vi "Create Host String.vi"(8 "Redirect Endpoint":string, 9 "URL Prefix":string, 10 "Region":string, 11 "AWS Service":string) -> (3 "Host String":string)   [LabVIEW 2015, in "NI_AWS_Core.lvclass"]
uses:
  NI_AWS_Core.lvclass
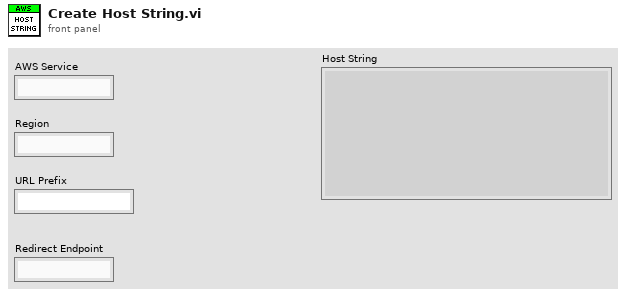
[diagram p1: front panel]
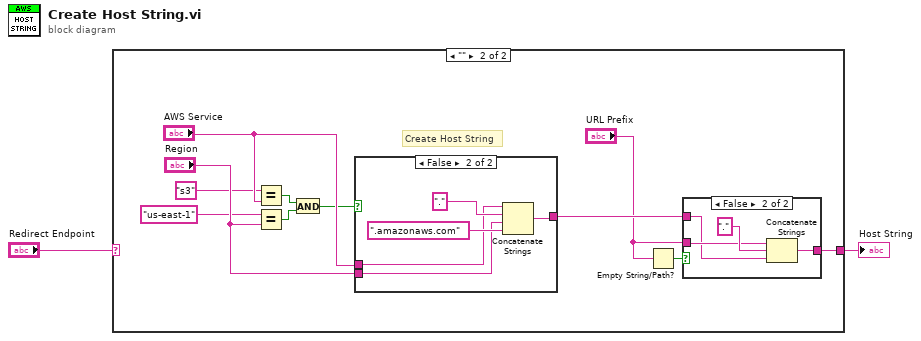
[diagram p0: block diagram]
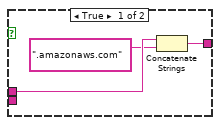
[diagram p4: hidden frame]
diagram:
  n1 = case shown="\"\"" "Redirect Endpoint" {
    selector: "Redirect Endpoint" -> [w3 _]
    tunnel: [w3 w4] -> w2
    frame Default {
    }
    frame "" {
      # "Create Host String"
      n2 = Equal?(x="s3", y="AWS Service") -> (x = y?=w5:bool)
      n3 = Equal?(x="us-east-1", y="Region") -> (x = y?=w7:bool)
      n4 = And(x=w5, y=w7) -> (x .and. y?=w9:bool)
      n5 = case shown="False" w9 {
        tunnel: [w22 w27] -> w14
        tunnel: "AWS Service" -> [w21 w23]
        tunnel: "Region" -> [_ w24]
        frame True {
          n6 = Concatenate Strings(w21, ".amazonaws.com" ("string")) -> (w22:string)
        }
        frame False {
          n7 = Concatenate Strings(w23, "." ("string"), w24, ".amazonaws.com" ("string")) -> (w27:string)
        }
      }
      n8 = Empty String/Path?(string/path="URL Prefix") -> (empty?=w12:bool)
      n9 = case shown="False" w12 {
        tunnel: [w15 w19] -> w4
        tunnel: "URL Prefix" -> [_ w17]
        tunnel: w14 -> [w15 w16]
        frame True {
        }
        frame False {
          n10 = Concatenate Strings(w17, "." ("string"), w16) -> (w19:string)
        }
      }
    }
  }
  "Host String" <- w2
